vi "GxSingleCam.vi"() -> ()   [LabVIEW 2013]
uses:
  GxLVLib/GxLVlib.lvlib
  F:/GxILibrary/Labview/trunk/private/dev/src/C#/x86/GxLVLib/dll/GxIAPINET.dll
  private/dev/src/C#/x86/GxLVLib/dll/GxIAPINET.dll
  <vilib>/vision/Image Controls.llb/IMAQ Image.ctl
panel:
  out "Image":T1(plugin-control)
  out "是否退出":bool
  in  "图片存储路径":path
  in  "保存图片":bool
  in  "Image Src":T1
  out "采集回调":refnum<k27>
  out "是否支持白平衡":bool
  out "采集状态":bool
  out "设备状态":bool
  in  "IGxFactory":refnum<k24>
  in  "安全退出":bool
  in  "IGxStream":refnum<k24>
  in  "IGxDevice":refnum<k24>
  out "error out":errorcluster
  in  "发送软触发":bool
  in  "自动白平衡":string(combo)
  in  "增益":dbl format="%#_6f"
  in  "曝光时间":dbl
  in  "触发源":string(combo)
  in  "触发模式":string(combo)
  in  "停止采集":bool
  in  "开始采集":bool
  in  "关闭设备":bool
  in  "打开设备":bool
  # "触发模式"
  # "触发源"
  # "软触发"
  # "曝光时间(us)"
  # "增益(dB)"
  # "自动白平衡"
  # "保存图片"
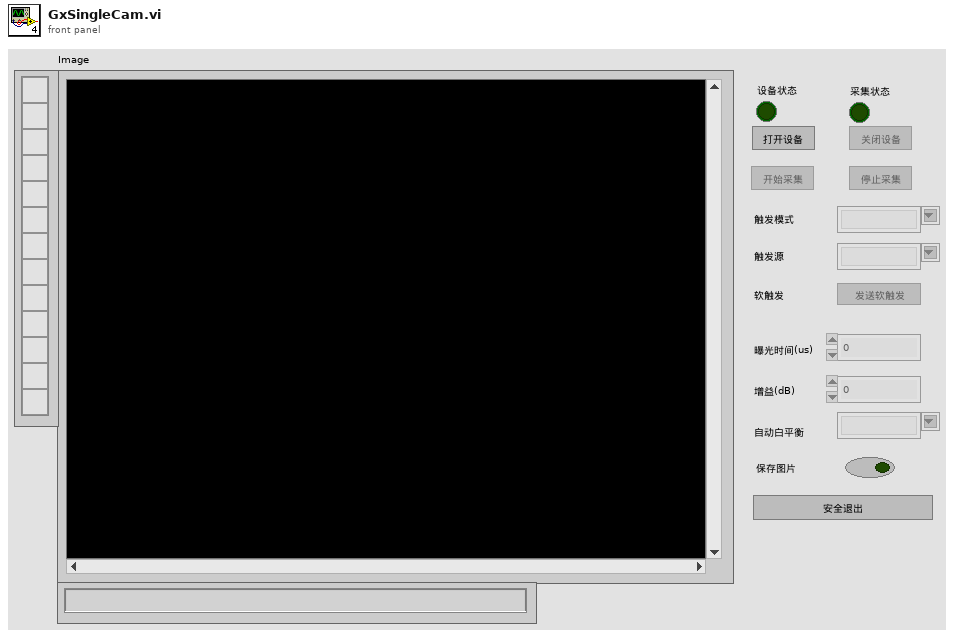
[diagram p1: front panel]
types:
  T1 = typedef "IMAQ Image.ctl" = refnum<image>
  T2 = typedef "Semaphore RefNum" = refnum<k1>
  T3 = enum8{"Enabled", "Disabled", "Disabled and Grayed Out"}
  T4 = typedef "Image Type" = u32
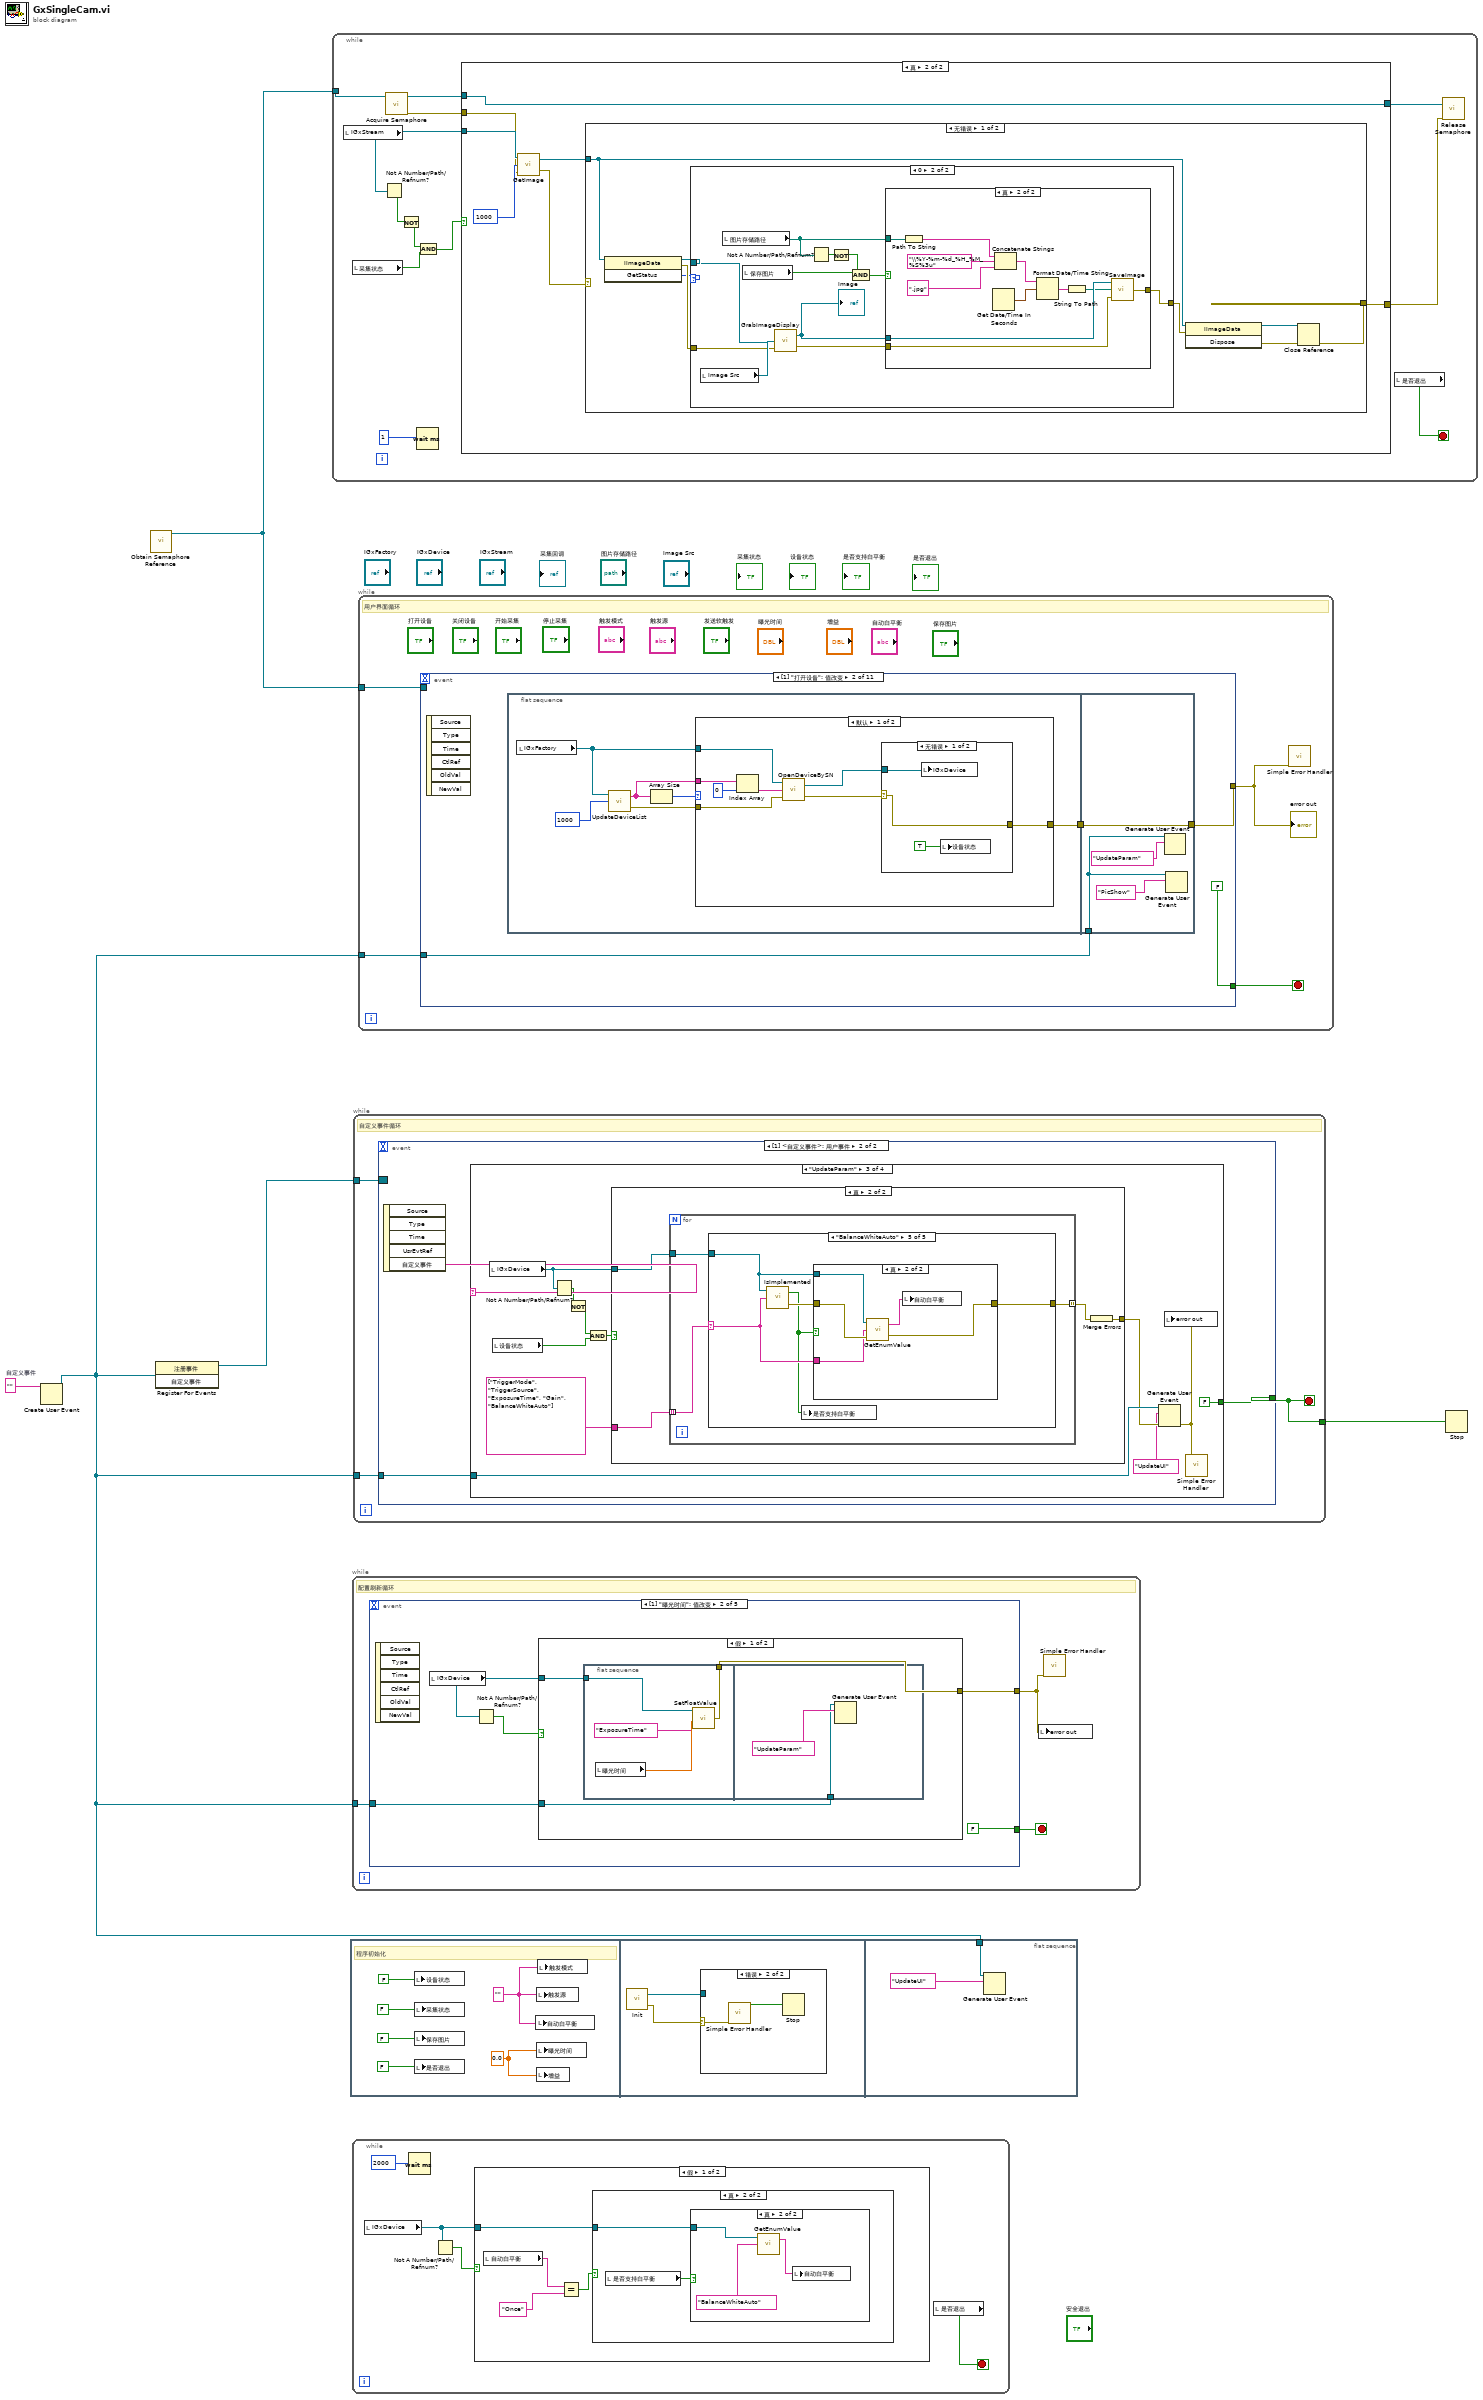
[diagram p0: block diagram]
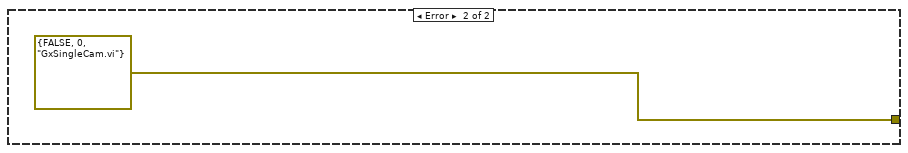
[diagram p5: hidden frame]
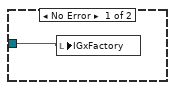
[diagram p9: hidden frame]
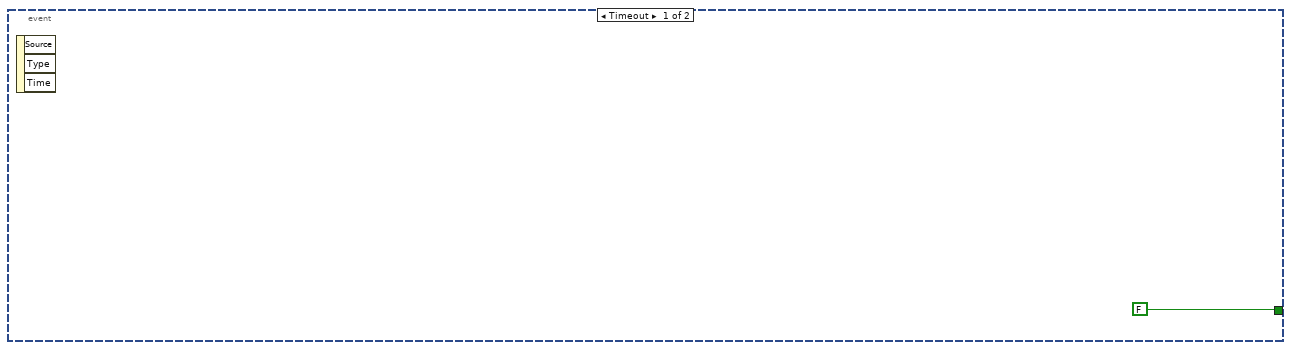
[diagram p10: hidden frame]
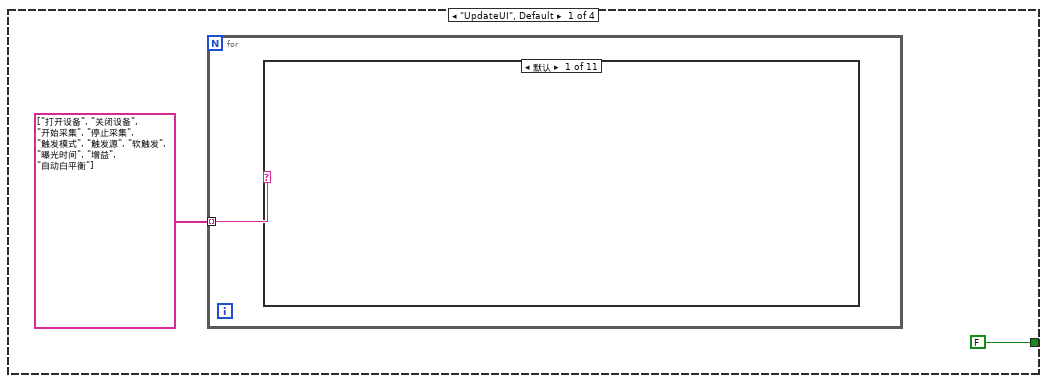
[diagram p11: hidden frame]
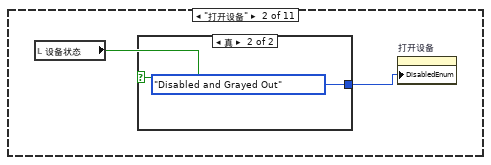
[diagram p12: hidden frame]
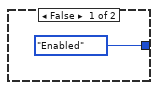
[diagram p13: hidden frame]
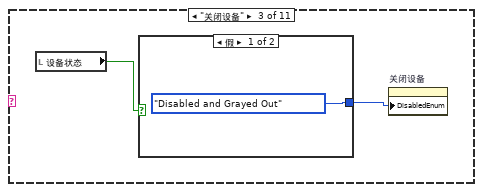
[diagram p14: hidden frame]
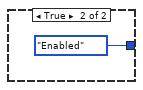
[diagram p15: hidden frame]
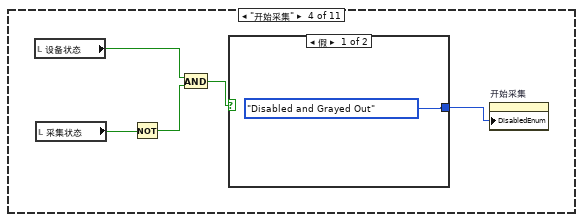
[diagram p16: hidden frame]
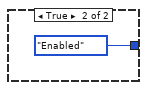
[diagram p17: hidden frame]
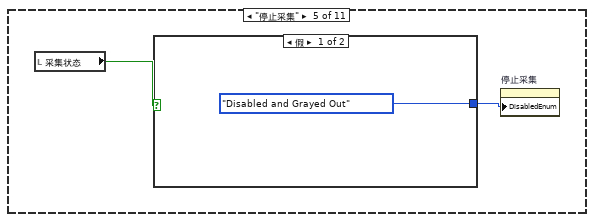
[diagram p18: hidden frame]
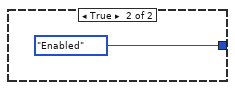
[diagram p19: hidden frame]
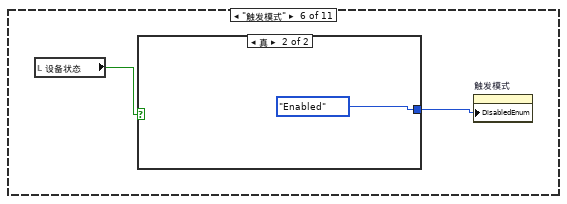
[diagram p20: hidden frame]
diagram:
  w5 = ""  # 自定义事件
  n1 = Create User Event(user event datatype=w5) -> (user event=w2:refnum<user-event>)  [unwired: 1 in, 1 out]
  n2 = call <vilib>:"Obtain Semaphore Reference.vi"() -> ("semaphore"=w1:T2)  [unwired: 5 in, 2 out]
  n3 = register-events(w2) -> (reference out=w4:refnum<event-registration>)  [unwired: 2 in, 1 out]
  n4 = while {
    tunnel: w1 -> [w10]
    stop <- w17 stop-if-true
    n5 = local read "IGxStream"() -> (w16:refnum<k24>)
    n6 = local read "采集状态"() -> (w13:bool)
    n7 = Not A Number/Path/Refnum?(number/path/refnum=w16) -> (NaN/Path/Refnum?=w15:bool)
    n8 = call <vilib>:"Acquire Semaphore.vi"("semaphore"=w10) -> ("error out"=w7:errorcluster, "semaphore out"=w9:T2)  [unwired: 4 in, 1 out]
    n9 = Not(x=w15) -> (.not. x?=w14:bool)
    n10 = Wait (ms)(milliseconds to wait=1) -> ()  [unwired: 1 out]
    n11 = And(x=w14, y=w13) -> (x .and. y?=w12:bool)
    n12 = case shown="真" w12 {
      tunnel: w16 -> [_ w26]
      tunnel: [w18 w24] -> w8
      tunnel: w9 -> [w18 w24]
      tunnel: w7 -> [w19 w23]
      tunnel: [w19 w20] -> w6
      frame False {
      }
      frame True {
        n13 = call "GetImage.vi"("error in (no error)"=w23, "Time out"=1000, "IGxStream"=w26) -> ("error out"=w22:errorcluster, "IImageData"=w21:refnum<k24>)
        n14 = case shown="无错误" w22 {
          tunnel: w21 -> [w30 _]
          tunnel: [w28 errorcluster {FALSE, 0, "GxSingleCam.vi"}] -> w20
          frame No Error {
            n15 = invoke class="IImageData" method="GetStatus"(reference=w30) -> (reference out=w33:refnum<k24>, error out=w34:errorcluster, "GetStatus"=w32:i32)  [unwired: 2 in]
            n16 = case shown="0" w32 {
              tunnel: [w35 w40] -> w31
              tunnel: w33 -> [_ w37]
              tunnel: w34 -> [w35 w38]
              frame Default {
              }
              frame 0 {
                n17 = local read "Image Src"() -> (w41:T1)
                n18 = local read "图片存储路径"() -> (w39:path)
                n19 = local read "保存图片"() -> (w44:bool)
                n20 = call "GrabImageDisplay.vi"("error in (no error)"=w38, "Image Src"=w41, "IBaseData"=w37) -> ("error out"=w46:errorcluster, "Image out"=w36:T1)
                "Image" <- w36
                n21 = Not A Number/Path/Refnum?(number/path/refnum=w39) -> (NaN/Path/Refnum?=w42:bool)
                n22 = Not(x=w42) -> (.not. x?=w43:bool)
                n23 = And(x=w44, y=w43) -> (x .and. y?=w45:bool)
                n24 = case shown="真" w45 {
                  tunnel: w39 -> [_ w54]
                  tunnel: w36 -> [_ w53]
                  tunnel: w46 -> [w47 w51]
                  tunnel: [w47 w50] -> w40
                  frame False {
                  }
                  frame True {
                    n25 = Path To String(path=w54) -> (string=w55:string)
                    n26 = Get Date/Time In Seconds() -> (seconds since 1Jan1904=w57:timestamp)
                    n27 = Concatenate Strings(w55, "\\%Y-%m-%d_%H_%M_%S%3u", ".jpg") -> (w56:string)
                    n28 = Format Date/Time String(time format string (%c)=w56, seconds (now)=w57) -> (date/time string=w58:string)  [unwired: 1 in]
                    n29 = String To Path(string=w58) -> (path=w52:path)
                    n30 = call "SaveImage.vi"("error in (no error)"=w51, "Path"=w52, "Image Src"=w53) -> ("error out"=w50:errorcluster)
                  }
                }
              }
            }
            n31 = invoke class="IImageData" method="Dispose"(reference=w30, error in=w31) -> (reference out=w27:refnum<k24>, error out=w29:errorcluster)  [unwired: 1 in, 1 out]
            n32 = Close Reference(reference=w27, error in (no error)=w29) -> (error out=w28:errorcluster)
          }
          frame Error {
          }
        }
      }
    }
    n33 = local read "是否退出"() -> (w17:bool)
    n34 = call <vilib>:"Release Semaphore.vi"("error in (no error)"=w6, "semaphore"=w8) -> ()  [unwired: 4 in, 2 out]
  }
  n35 = flat-sequence {
    tunnel: w2 -> [w71]
    frame #0 {
      w62 = 0.0
      w63 = ""
      # "程序初始化"
      n36 = local write "设备状态"(FALSE) -> ()
      n37 = local write "采集状态"(FALSE) -> ()
      n38 = local write "保存图片"(FALSE) -> ()
      n39 = local write "是否退出"(FALSE) -> ()
      n40 = local write "自动白平衡"(w63) -> ()
      n41 = local write "触发源"(w63) -> ()
      n42 = local write "曝光时间"(w62) -> ()
      n43 = local write "增益"(w62) -> ()
      n44 = local write "触发模式"(w63) -> ()
    }
    frame #1 {
      n45 = call "Init.vi"() -> ("IGxFactory"=w67:refnum<k24>, "error out"=w66:errorcluster)  [unwired: 1 in]
      n46 = case shown="错误" w66 {
        selector: w66 -> [_ w69]
        tunnel: w67 -> [w68 _]
        frame No Error {
          n47 = local write "IGxFactory"(w68) -> ()
        }
        frame Error {
          n48 = call <vilib>:"Simple Error Handler.vi"("error in (no error)"=w69) -> ("error?"=w70:bool)  [unwired: 4 in, 4 out]
          n49 = Stop(stop? (T)=w70) -> ()
        }
      }
    }
    frame #2 {
      n50 = Generate User Event(user event=w71, event data cluster="UpdateUI") -> ()  [unwired: 2 in, 2 out]
    }
  }
  n51 = while {
    tunnel: w2 -> [w73]
    stop <- w75 stop-if-true
    # "配置刷新循环"
    n52 = event shown="[1] \"曝光时间\": 值改变" {
      selector: _ -> [_ _ _ _ _]
      dyn-events: _ -> [_ _ _ _ _]
      timeout: _ -> [_ _ _ _ _]
      tunnel: [errorcluster {FALSE, 0, ""} w80 w95 w110 errorcluster {"status"=FALSE, "code"=0, "source"=""} ("错误常量")] -> w74
      tunnel: [FALSE FALSE FALSE FALSE TRUE] -> w75
      tunnel: w73 -> [_ w78 w93 w108 _]
      event Timeout {
        n53 = event-data() -> ()  [unwired: 1 in, 3 out]
      }
      event "曝光时间": Value Change {
        n54 = event-data() -> ()  [unwired: 1 in, 6 out]
        n55 = local read "IGxDevice"() -> (w81:refnum<k24>)
        n56 = Not A Number/Path/Refnum?(number/path/refnum=w81) -> (NaN/Path/Refnum?=w82:bool)
        n57 = case shown="假" w82 {
          tunnel: w81 -> [w85 _]
          tunnel: [w84 errorcluster {TRUE, 5000, "GxSingleCam.vi"}] -> w80
          tunnel: w78 -> [w83 _]
          frame False {
            n58 = flat-sequence {
              tunnel: w85 -> [w87]
              tunnel: [w86] -> w84
              tunnel: w83 -> [w90]
              frame #0 {
                n59 = local read "曝光时间"() -> (w89:dbl)
                n60 = call "SetFloatValue.vi"("Float Value"=w89, "Feature Name"="ExposureTime", "IGxDevice"=w87) -> ("error out"=w86:errorcluster)  [unwired: 1 in]
              }
              frame #1 {
                n61 = Generate User Event(user event=w90, event data cluster="UpdateParam") -> ()  [unwired: 2 in, 2 out]
              }
            }
          }
          frame True {
          }
        }
      }
      event "增益": Value Change {
        n62 = event-data() -> ()  [unwired: 1 in, 6 out]
        n63 = local read "IGxDevice"() -> (w97:refnum<k24>)
        n64 = Not A Number/Path/Refnum?(number/path/refnum=w97) -> (NaN/Path/Refnum?=w96:bool)
        n65 = case shown="真" w96 {
          tunnel: w97 -> [w100 _]
          tunnel: [w99 errorcluster {TRUE, 0, "设备句柄无效"}] -> w95
          tunnel: w93 -> [w98 _]
          frame False {
            n66 = flat-sequence {
              tunnel: w100 -> [w102]
              tunnel: [w101] -> w99
              tunnel: w98 -> [w106]
              frame #0 {
                n67 = local read "增益"() -> (w104:dbl)
                n68 = call "SetFloatValue.vi"("Float Value"=w104, "Feature Name"="Gain", "IGxDevice"=w102) -> ("error out"=w101:errorcluster)  [unwired: 1 in]
              }
              frame #1 {
                n69 = Generate User Event(user event=w106, event data cluster="UpdateParam") -> ()  [unwired: 2 in, 2 out]
              }
            }
          }
          frame True {
          }
        }
      }
      event "自动白平衡": Value Change {
        n70 = event-data() -> ()  [unwired: 1 in, 6 out]
        n71 = local read "IGxDevice"() -> (w111:refnum<k24>)
        n72 = Not A Number/Path/Refnum?(number/path/refnum=w111) -> (NaN/Path/Refnum?=w112:bool)
        n73 = case shown="假" w112 {
          tunnel: w111 -> [w115 _]
          tunnel: [w114 errorcluster {TRUE, 0, "设备句柄无效"}] -> w110
          tunnel: w108 -> [w113 _]
          frame False {
            n74 = flat-sequence {
              tunnel: w115 -> [w117]
              tunnel: [w116] -> w114
              tunnel: w113 -> [w120]
              frame #0 {
                n75 = local read "自动白平衡"() -> (w119:string)
                n76 = call "SetEnumValue.vi"("Enum Value"=w119, "Feature Name"="BalanceWhiteAuto", "IGxDevice"=w117) -> ("error out"=w116:errorcluster)  [unwired: 1 in]
              }
              frame #1 {
                n77 = Generate User Event(user event=w120, event data cluster="UpdateParam") -> ()  [unwired: 2 in, 2 out]
              }
            }
          }
          frame True {
          }
        }
      }
      event "安全退出": Value Change {
        n78 = event-data() -> ()  [unwired: 1 in, 6 out]
      }
    }
    n79 = local write "error out"(w74) -> ()
    n80 = call <vilib>:"Simple Error Handler.vi"("error in (no error)"=w74) -> ()  [unwired: 4 in, 5 out]
  }
  n81 = while {
    stop <- w125 stop-if-true
    n82 = local read "IGxDevice"() -> (w127:refnum<k24>)
    n83 = Wait (ms)(milliseconds to wait=2000) -> ()  [unwired: 1 out]
    n84 = Not A Number/Path/Refnum?(number/path/refnum=w127) -> (NaN/Path/Refnum?=w126:bool)
    n85 = case shown="假" w126 {
      tunnel: w127 -> [w132 _]
      frame False {
        n86 = local read "自动白平衡"() -> (w130:string)
        n87 = Equal?(x=w130, y="Once") -> (x = y?=w129:bool)
        n88 = case shown="真" w129 {
          tunnel: w132 -> [_ w133]
          frame False {
          }
          frame True {
            n89 = local read "是否支持白平衡"() -> (w134:bool)
            n90 = case shown="真" w134 {
              tunnel: w133 -> [_ w137]
              frame False {
              }
              frame True {
                n91 = call "GetEnumValue.vi"("Feature Name"="BalanceWhiteAuto", "IGxDevice"=w137) -> ("Enum Value"=w135:string)  [unwired: 1 in, 1 out]
                n92 = local write "自动白平衡"(w135) -> ()
              }
            }
          }
        }
      }
      frame True {
      }
    }
    n93 = local read "是否退出"() -> (w125:bool)
  }
  n94 = while {
    tunnel: w4 -> [w140]
    tunnel: w2 -> [w139]
    tunnel: [w138] -> w3
    stop <- w138 stop-if-true
    # "自定义事件循环"
    n95 = event shown="[1] <自定义事件>: 用户事件" {
      selector: w140 -> [_ _]
      dyn-events: _ -> [_ _]
      timeout: _ -> [_ _]
      tunnel: [FALSE w142] -> w138
      tunnel: w139 -> [_ w143]
      event Timeout {
        n96 = event-data() -> ()  [unwired: 1 in, 3 out]
      }
      event User Event {
        n97 = event-data() -> ("自定义事件"=w144:string)  [unwired: 1 in, 4 out]
        n98 = case shown="\"UpdateParam\"" w144 {
          tunnel: w143 -> [_ _ w275 _]
          tunnel: [FALSE TRUE FALSE FALSE] -> w142
          frame "UpdateUI", Default {
            n99 = for {
              tunnel: string[] ["打开设备", "关闭设备", "开始采集", "停止采集", "触发模式", "触发源", "软触发", "曝光时间", "增益", "自动白平衡"] -> [w147] mode=indexing
              n100 = case shown="默认" w147 {
                frame Default {
                }
                frame "打开设备" {
                  n101 = local read "设备状态"() -> (w149:bool)
                  n102 = case shown="真" w149 {
                    tunnel: [T3."Enabled" ("禁用") T3."Disabled and Grayed Out" ("禁用")] -> w148
                    frame False {
                    }
                    frame True {
                    }
                  }
                  n103 = property on="打开设备" class="Bool"("DisabledEnum"=w148) -> ()  [unwired: 2 in, 2 out]
                }
                frame "关闭设备" {
                  n104 = local read "设备状态"() -> (w153:bool)
                  n105 = case shown="假" w153 {
                    tunnel: [T3."Disabled and Grayed Out" ("禁用") T3."Enabled" ("禁用")] -> w152
                    frame False {
                    }
                    frame True {
                    }
                  }
                  n106 = property on="关闭设备" class="Bool"("DisabledEnum"=w152) -> ()  [unwired: 2 in, 2 out]
                }
                frame "开始采集" {
                  n107 = local read "设备状态"() -> (w159:bool)
                  n108 = local read "采集状态"() -> (w160:bool)
                  n109 = Not(x=w160) -> (.not. x?=w158:bool)
                  n110 = And(x=w159, y=w158) -> (x .and. y?=w157:bool)
                  n111 = case shown="假" w157 {
                    tunnel: [T3."Disabled and Grayed Out" ("禁用") T3."Enabled" ("禁用")] -> w156
                    frame False {
                    }
                    frame True {
                    }
                  }
                  n112 = property on="开始采集" class="Bool"("DisabledEnum"=w156) -> ()  [unwired: 2 in, 2 out]
                }
                frame "停止采集" {
                  n113 = local read "采集状态"() -> (w164:bool)
                  n114 = case shown="假" w164 {
                    tunnel: [T3."Disabled and Grayed Out" ("禁用") T3."Enabled" ("禁用")] -> w163
                    frame False {
                    }
                    frame True {
                    }
                  }
                  n115 = property on="停止采集" class="Bool"("DisabledEnum"=w163) -> ()  [unwired: 2 in, 2 out]
                }
                frame "触发模式" {
                  n116 = local read "设备状态"() -> (w168:bool)
                  n117 = case shown="真" w168 {
                    tunnel: [T3."Disabled and Grayed Out" ("禁用") T3."Enabled" ("禁用")] -> w167
                    frame False {
                    }
                    frame True {
                    }
                  }
                  n118 = property on="触发模式" class="CmbBox"("DisabledEnum"=w167) -> ()  [unwired: 2 in, 2 out]
                }
                frame "触发源" {
                  n119 = local read "设备状态"() -> (w174:bool)
                  n120 = local read "触发模式"() -> (w176:string)
                  n121 = Equal?(x=w176, y="On") -> (x = y?=w173:bool)
                  n122 = And(x=w174, y=w173) -> (x .and. y?=w172:bool)
                  n123 = case shown="假" w172 {
                    tunnel: [T3."Disabled and Grayed Out" ("禁用") T3."Enabled" ("禁用")] -> w171
                    frame False {
                    }
                    frame True {
                    }
                  }
                  n124 = property on="触发源" class="CmbBox"("DisabledEnum"=w171) -> ()  [unwired: 2 in, 2 out]
                }
                frame "软触发" {
                  n125 = local read "设备状态"() -> (w181:bool)
                  n126 = local read "采集状态"() -> (w180:bool)
                  n127 = local read "触发模式"() -> (w190:string)
                  n128 = local read "触发源"() -> (w188:string)
                  n129 = Equal?(x=w190, y="On") -> (x = y?=w186:bool)
                  n130 = Equal?(x=w188, y="Software") -> (x = y?=w185:bool)
                  n131 = And(x=w181, y=w180) -> (x .and. y?=w179:bool)
                  n132 = And(x=w186, y=w185) -> (x .and. y?=w184:bool)
                  n133 = And(x=w179, y=w184) -> (x .and. y?=w183:bool)
                  n134 = case shown="真" w183 {
                    tunnel: [T3."Disabled and Grayed Out" ("禁用") T3."Enabled" ("禁用")] -> w182
                    frame False {
                    }
                    frame True {
                    }
                  }
                  n135 = property on="发送软触发" class="Bool"("DisabledEnum"=w182) -> ()  [unwired: 2 in, 2 out]
                }
                frame "曝光时间" {
                  n136 = local read "设备状态"() -> (w194:bool)
                  n137 = case shown="假" w194 {
                    tunnel: [T3."Disabled and Grayed Out" ("禁用") T3."Enabled" ("禁用")] -> w193
                    frame False {
                    }
                    frame True {
                    }
                  }
                  n138 = property on="曝光时间" class="DigNum (严格)"("DisabledEnum"=w193) -> ()  [unwired: 2 in, 2 out]
                }
                frame "增益" {
                  n139 = local read "设备状态"() -> (w198:bool)
                  n140 = case shown="真" w198 {
                    tunnel: [T3."Disabled and Grayed Out" ("禁用") T3."Enabled" ("禁用")] -> w197
                    frame False {
                    }
                    frame True {
                    }
                  }
                  n141 = property on="增益" class="DigNum (严格)"("DisabledEnum"=w197) -> ()  [unwired: 2 in, 2 out]
                }
                frame "自动白平衡" {
                  n142 = local read "是否支持白平衡"() -> (w204:bool)
                  n143 = local read "设备状态"() -> (w203:bool)
                  n144 = And(x=w203, y=w204) -> (x .and. y?=w202:bool)
                  n145 = case shown="真" w202 {
                    tunnel: [T3."Disabled and Grayed Out" ("禁用") T3."Enabled" ("禁用")] -> w201
                    frame False {
                    }
                    frame True {
                    }
                  }
                  n146 = property on="自动白平衡" class="CmbBox"("DisabledEnum"=w201) -> ()  [unwired: 2 in, 2 out]
                }
              }
            }
          }
          frame "Quit" {
            n147 = for {
              tunnel: string[] ["打开设备", "关闭设备", "开始采集", "停止采集", "触发模式", "触发源", "软触发", "曝光时间", "增益", "自动白平衡"] -> [w211] mode=indexing
              n148 = case shown="\"停止采集\"" w211 {
                frame Default {
                }
                frame "打开设备" {
                  n149 = local read "设备状态"() -> (w213:bool)
                  n150 = case shown="真" w213 {
                    tunnel: [T3."Enabled" ("禁用") T3."Disabled and Grayed Out" ("禁用")] -> w212
                    frame False {
                    }
                    frame True {
                    }
                  }
                  n151 = property on="打开设备" class="Bool"("DisabledEnum"=w212) -> ()  [unwired: 2 in, 2 out]
                }
                frame "关闭设备" {
                  n152 = local read "设备状态"() -> (w217:bool)
                  n153 = case shown="假" w217 {
                    tunnel: [T3."Disabled and Grayed Out" ("禁用") T3."Enabled" ("禁用")] -> w216
                    frame False {
                    }
                    frame True {
                    }
                  }
                  n154 = property on="关闭设备" class="Bool"("DisabledEnum"=w216) -> ()  [unwired: 2 in, 2 out]
                }
                frame "开始采集" {
                  n155 = local read "设备状态"() -> (w223:bool)
                  n156 = local read "采集状态"() -> (w224:bool)
                  n157 = Not(x=w224) -> (.not. x?=w222:bool)
                  n158 = And(x=w223, y=w222) -> (x .and. y?=w221:bool)
                  n159 = case shown="假" w221 {
                    tunnel: [T3."Disabled and Grayed Out" ("禁用") T3."Enabled" ("禁用")] -> w220
                    frame False {
                    }
                    frame True {
                    }
                  }
                  n160 = property on="开始采集" class="Bool"("DisabledEnum"=w220) -> ()  [unwired: 2 in, 2 out]
                }
                frame "停止采集" {
                  n161 = local read "采集状态"() -> (w228:bool)
                  n162 = case shown="假" w228 {
                    tunnel: [T3."Disabled and Grayed Out" ("禁用") T3."Enabled" ("禁用")] -> w227
                    frame False {
                    }
                    frame True {
                    }
                  }
                  n163 = property on="停止采集" class="Bool"("DisabledEnum"=w227) -> ()  [unwired: 2 in, 2 out]
                }
                frame "触发模式" {
                  n164 = local read "设备状态"() -> (w232:bool)
                  n165 = case shown="真" w232 {
                    tunnel: [T3."Disabled and Grayed Out" ("禁用") T3."Enabled" ("禁用")] -> w231
                    frame False {
                    }
                    frame True {
                    }
                  }
                  n166 = property on="触发模式" class="CmbBox"("DisabledEnum"=w231) -> ()  [unwired: 2 in, 2 out]
                }
                frame "触发源" {
                  n167 = local read "设备状态"() -> (w238:bool)
                  n168 = local read "触发模式"() -> (w240:string)
                  n169 = Equal?(x=w240, y="On") -> (x = y?=w237:bool)
                  n170 = And(x=w238, y=w237) -> (x .and. y?=w236:bool)
                  n171 = case shown="假" w236 {
                    tunnel: [T3."Disabled and Grayed Out" ("禁用") T3."Enabled" ("禁用")] -> w235
                    frame False {
                    }
                    frame True {
                    }
                  }
                  n172 = property on="触发源" class="CmbBox"("DisabledEnum"=w235) -> ()  [unwired: 2 in, 2 out]
                }
                frame "软触发" {
                  n173 = local read "设备状态"() -> (w245:bool)
                  n174 = local read "采集状态"() -> (w244:bool)
                  n175 = local read "触发模式"() -> (w254:string)
                  n176 = local read "触发源"() -> (w252:string)
                  n177 = Equal?(x=w254, y="On") -> (x = y?=w250:bool)
                  n178 = Equal?(x=w252, y="Software") -> (x = y?=w249:bool)
                  n179 = And(x=w245, y=w244) -> (x .and. y?=w243:bool)
                  n180 = And(x=w250, y=w249) -> (x .and. y?=w248:bool)
                  n181 = And(x=w243, y=w248) -> (x .and. y?=w247:bool)
                  n182 = case shown="真" w247 {
                    tunnel: [T3."Disabled and Grayed Out" ("禁用") T3."Enabled" ("禁用")] -> w246
                    frame False {
                    }
                    frame True {
                    }
                  }
                  n183 = property on="发送软触发" class="Bool"("DisabledEnum"=w246) -> ()  [unwired: 2 in, 2 out]
                }
                frame "曝光时间" {
                  n184 = local read "设备状态"() -> (w258:bool)
                  n185 = case shown="假" w258 {
                    tunnel: [T3."Disabled and Grayed Out" ("禁用") T3."Enabled" ("禁用")] -> w257
                    frame False {
                    }
                    frame True {
                    }
                  }
                  n186 = property on="曝光时间" class="DigNum (严格)"("DisabledEnum"=w257) -> ()  [unwired: 2 in, 2 out]
                }
                frame "增益" {
                  n187 = local read "设备状态"() -> (w262:bool)
                  n188 = case shown="真" w262 {
                    tunnel: [T3."Disabled and Grayed Out" ("禁用") T3."Enabled" ("禁用")] -> w261
                    frame False {
                    }
                    frame True {
                    }
                  }
                  n189 = property on="增益" class="DigNum (严格)"("DisabledEnum"=w261) -> ()  [unwired: 2 in, 2 out]
                }
                frame "自动白平衡" {
                  n190 = local read "是否支持白平衡"() -> (w268:bool)
                  n191 = local read "设备状态"() -> (w267:bool)
                  n192 = And(x=w267, y=w268) -> (x .and. y?=w266:bool)
                  n193 = case shown="真" w266 {
                    tunnel: [T3."Disabled and Grayed Out" ("禁用") T3."Enabled" ("禁用")] -> w265
                    frame False {
                    }
                    frame True {
                    }
                  }
                  n194 = property on="自动白平衡" class="CmbBox"("DisabledEnum"=w265) -> ()  [unwired: 2 in, 2 out]
                }
              }
            }
            n195 = local read "IGxFactory"() -> (w207:refnum<k24>)
            n196 = call "UnInit.vi"("IGxFactory"=w207) -> ("error out"=w208:errorcluster)  [unwired: 1 in]
            n197 = Close Reference(reference=w207, error in (no error)=w208) -> ()  [unwired: 1 out]
          }
          frame "UpdateParam" {
            n198 = local read "IGxDevice"() -> (w277:refnum<k24>)
            n199 = local read "设备状态"() -> (w281:bool)
            n200 = Not A Number/Path/Refnum?(number/path/refnum=w277) -> (NaN/Path/Refnum?=w278:bool)
            n201 = Not(x=w278) -> (.not. x?=w280:bool)
            n202 = And(x=w280, y=w281) -> (x .and. y?=w279:bool)
            n203 = case shown="真" w279 {
              tunnel: [errorcluster {FALSE, 0, ""} w283] -> w274
              tunnel: string[] ["TriggerMode", "TriggerSource", "ExposureTime", "Gain", "BalanceWhiteAuto"] -> [_ w286]
              tunnel: w277 -> [_ w285]
              frame False {
              }
              frame True {
                n204 = for {
                  tunnel: w286 -> [w289] mode=indexing
                  tunnel: w285 -> [w288]
                  tunnel: [w287] -> w284 mode=indexing
                  n205 = case shown="\"BalanceWhiteAuto\"" w289 {
                    selector: w289 -> [w292 w296 w300 w304 w307]
                    tunnel: w288 -> [w293 w297 w301 w305 w308]
                    tunnel: [w290 w294 w298 w302 w310] -> w287
                    frame "TriggerMode", Default {
                      n206 = call "GetEnumValue.vi"("Feature Name"=w292, "IGxDevice"=w293) -> ("error out"=w290:errorcluster, "Enum Value"=w291:string)  [unwired: 1 in]
                      n207 = local write "触发模式"(w291) -> ()
                    }
                    frame "TriggerSource" {
                      n208 = call "GetEnumValue.vi"("Feature Name"=w296, "IGxDevice"=w297) -> ("error out"=w294:errorcluster, "Enum Value"=w295:string)  [unwired: 1 in]
                      n209 = local write "触发源"(w295) -> ()
                    }
                    frame "ExposureTime" {
                      n210 = call "GetFloatValue.vi"("Feature Name"=w300, "IGxDevice"=w301) -> ("error out"=w298:errorcluster, "Float Value"=w299:dbl)  [unwired: 1 in]
                      n211 = local write "曝光时间"(w299) -> ()
                    }
                    frame "Gain" {
                      n212 = call "GetFloatValue.vi"("Feature Name"=w304, "IGxDevice"=w305) -> ("error out"=w302:errorcluster, "Float Value"=w303:dbl)  [unwired: 1 in]
                      n213 = local write "增益"(w303) -> ()
                    }
                    frame "BalanceWhiteAuto" {
                      n214 = call "IsImplemented.vi"("Feature Name"=w307, "IGxDevice"=w308) -> ("error out"=w309:errorcluster, "IsImplement"=w306:bool)  [unwired: 1 in]
                      n215 = local write "是否支持白平衡"(w306) -> ()
                      n216 = case shown="真" w306 {
                        tunnel: [w311 w315] -> w310
                        tunnel: w309 -> [w311 w316]
                        tunnel: w308 -> [_ w313]
                        tunnel: w307 -> [_ w312]
                        frame False {
                        }
                        frame True {
                          n217 = call "GetEnumValue.vi"("error in (no error)"=w316, "Feature Name"=w312, "IGxDevice"=w313) -> ("error out"=w315:errorcluster, "Enum Value"=w314:string)
                          n218 = local write "自动白平衡"(w314) -> ()
                        }
                      }
                    }
                  }
                }
                n219 = Merge Errors(w284) -> (w283:errorcluster)
              }
            }
            n220 = Generate User Event(user event=w275, event data cluster="UpdateUI", error in=w274) -> (error out=w273:errorcluster)  [unwired: 1 in, 1 out]
            n221 = local write "error out"(w273) -> ()
            n222 = call <vilib>:"Simple Error Handler.vi"("error in (no error)"=w273) -> ()  [unwired: 4 in, 5 out]
          }
          frame "PicShow" {
            n223 = local read "IGxDevice"() -> (w319:refnum<k24>)
            n224 = local read "设备状态"() -> (w323:bool)
            n225 = Not A Number/Path/Refnum?(number/path/refnum=w319) -> (NaN/Path/Refnum?=w320:bool)
            n226 = Not(x=w320) -> (.not. x?=w322:bool)
            n227 = And(x=w322, y=w323) -> (x .and. y?=w321:bool)
            n228 = case shown="真" w321 {
              tunnel: [errorcluster {FALSE, 0, ""} errorcluster {FALSE, 0, ""}] -> w317
              tunnel: w319 -> [_ w329]
              frame False {
              }
              frame True {
                n229 = call "IsImplemented.vi"("Feature Name"="PixelColorFilter", "IGxDevice"=w329) -> ("IsImplement"=w331:bool)  [unwired: 1 in, 1 out]
                n230 = case shown="真" w331 {
                  tunnel: w329 -> [_ w338]
                  tunnel: [w332 w333] -> w326
                  frame False {
                    w332 = T4 0 items=["Grayscale (U8)", "Grayscale (I16)", "Grayscale (SGL)", "Complex (CSG)", "RGB (U32)", "HSL (U32)", "RGB (U64)", "Grayscale (U16)"] ("Image Type")
                  }
                  frame True {
                    n231 = call "GetEnumValue.vi"("Feature Name"="PixelColorFilter", "IGxDevice"=w338) -> ("Enum Value"=w336:string)  [unwired: 1 in, 1 out]
                    n232 = Equal?(x=w336, y="None") -> (x = y?=w334:bool)
                    n233 = case shown="假" w334 {
                      tunnel: [w339 w340] -> w333
                      frame False {
                        w339 = T4 4 items=["Grayscale (U8)", "Grayscale (I16)", "Grayscale (SGL)", "Complex (CSG)", "RGB (U32)", "HSL (U32)", "RGB (U64)", "Grayscale (U16)"] ("Image Type")
                      }
                      frame True {
                        w340 = T4 0 items=["Grayscale (U8)", "Grayscale (I16)", "Grayscale (SGL)", "Complex (CSG)", "RGB (U32)", "HSL (U32)", "RGB (U64)", "Grayscale (U16)"] ("Image Type")
                      }
                    }
                  }
                }
                n234 = call "IMAQ Create"("Image Name"="", "Image Type"=w326) -> ("New Image"=w327:T1)  [unwired: 3 in, 1 out]
                n235 = local write "Image Src"(w327) -> ()
              }
            }
            n236 = local write "error out"(w317) -> ()
            n237 = call <vilib>:"Simple Error Handler.vi"("error in (no error)"=w317) -> ()  [unwired: 4 in, 5 out]
          }
        }
      }
    }
  }
  n238 = while {
    tunnel: w2 -> [w344]
    tunnel: w1 -> [w341]
    stop <- w342 stop-if-true
    # "用户界面循环"
    n239 = event shown="[1] \"打开设备\": 值改变" {
      selector: _ -> [_ _ _ _ _ _ _ _ _ _ _]
      dyn-events: _ -> [_ _ _ _ _ _ _ _ _ _ _]
      timeout: _ -> [_ _ _ _ _ _ _ _ _ _ _]
      tunnel: [errorcluster {FALSE, 0, ""} w349 _ w410 w429 w452 w460 w467 _ _ _] -> w343
      tunnel: [FALSE FALSE FALSE FALSE FALSE FALSE FALSE FALSE FALSE TRUE TRUE] -> w342
      tunnel: w344 -> [_ w347 w377 w408 w430 w454 w461 w469 _ w487 w520]
      tunnel: w341 -> [_ _ w376 _ w436 _ _ _ _ w486 w519]
      event Timeout {
        n240 = event-data() -> ()  [unwired: 1 in, 3 out]
      }
      event "打开设备": Value Change {
        n241 = event-data() -> ()  [unwired: 1 in, 6 out]
        n242 = flat-sequence {
          tunnel: [w353] -> w348
          tunnel: [w375] -> w349
          tunnel: w348 -> [w375]
          tunnel: w347 -> [w372]
          frame #0 {
            n243 = local read "IGxFactory"() -> (w354:refnum<k24>)
            n244 = call "UpdateDeviceList.vi"("time out"=1000, "IGxFactory"=w354) -> ("error out"=w351:errorcluster, "DeviceSNList"=w352:string[])  [unwired: 1 in]
            n245 = Array Size(array=w352) -> (size(s)=w355:i32)
            n246 = case shown="默认" w355 {
              tunnel: w352 -> [w364 _]
              tunnel: w354 -> [w360 _]
              tunnel: [w359 w370] -> w353
              tunnel: w351 -> [w358 w371]
              frame Default {
                n247 = Index Array(array=w364, index=0) -> (element=w361:string)
                n248 = call "OpenDeviceBySN.vi"("error in (no error)"=w358, "SN"=w361, "IGxFactory"=w360) -> ("error out"=w357:errorcluster, "IGxDevice"=w362:refnum<k24>)
                n249 = case shown="无错误" w357 {
                  selector: w357 -> [w365 w368]
                  tunnel: w362 -> [w366 _]
                  tunnel: [w365 w368] -> w359
                  frame No Error {
                    n250 = local write "IGxDevice"(w366) -> ()
                    n251 = local write "设备状态"(TRUE) -> ()
                  }
                  frame Error {
                  }
                }
              }
              frame 0 {
                n252 = Merge Errors(w371, errorcluster {TRUE, 5001, "GxSingleCam.vi"}) -> (w370:errorcluster)
              }
            }
          }
          frame #1 {
            n253 = Generate User Event(user event=w372, event data cluster="UpdateParam") -> ()  [unwired: 2 in, 2 out]
            n254 = Generate User Event(user event=w372, event data cluster="PicShow") -> ()  [unwired: 2 in, 2 out]
          }
        }
      }
      event "关闭设备": Value Change {
        n255 = event-data() -> ()  [unwired: 1 in, 6 out]
        n256 = flat-sequence {
          tunnel: w376 -> [w381]
          tunnel: w377 -> [w406]
          frame #0 {
            n257 = local read "IGxStream"() -> (w385:refnum<k24>)
            n258 = local read "IGxDevice"() -> (w384:refnum<k24>)
            n259 = Not A Number/Path/Refnum?(number/path/refnum=w385) -> (NaN/Path/Refnum?=w386:bool)
            n260 = case shown="假" w386 {
              tunnel: w385 -> [w397 _]
              tunnel: w384 -> [w395 w405]
              tunnel: [w394 w405] -> w382
              tunnel: w381 -> [w392 _]
              frame False {
                n261 = call <vilib>:"Acquire Semaphore.vi"("semaphore"=w392) -> ("semaphore out"=w391:T2)  [unwired: 4 in, 2 out]
                n262 = flat-sequence {
                  tunnel: w397 -> [w399]
                  tunnel: [w400] -> w396
                  tunnel: w395 -> [w400]
                  tunnel: [w399] -> w393
                  tunnel: w391 -> [w398]
                  tunnel: [w398] -> w390
                  tunnel: w396 -> [w404]
                  tunnel: [w404] -> w394
                  tunnel: w393 -> [w402]
                  tunnel: [w401] -> w389
                  tunnel: w390 -> [w401]
                  frame #0 {
                    n263 = call "StopGrab.vi"("IGxStream"=w399, "IGxDevice"=w400) -> ()  [unwired: 1 in, 1 out]
                  }
                  frame #1 {
                    n264 = call "CloseStream.vi"("IGxStream"=w402) -> ("error out"=w403:errorcluster)  [unwired: 1 in]
                    n265 = Close Reference(reference=w402, error in (no error)=w403) -> ()  [unwired: 1 out]
                  }
                }
                n266 = call <vilib>:"Release Semaphore.vi"("semaphore"=w389) -> ()  [unwired: 5 in, 2 out]
              }
              frame True {
              }
            }
            n267 = local read "Image Src"() -> (w387:T1)
            n268 = call "CloseDevice.vi"("IGxDevice"=w382) -> ("error out"=w388:errorcluster)  [unwired: 1 in]
            n269 = Close Reference(reference=w382, error in (no error)=w388) -> (error out=w383:errorcluster)
            n270 = call "Imaq Dispose"("Image"=w387, "error in (no error)"=w383) -> ()  [unwired: 1 in, 4 out]
          }
          frame #1 {
            n271 = Generate User Event(user event=w406, event data cluster="UpdateUI") -> ()  [unwired: 2 in, 2 out]
          }
        }
        n272 = local write "采集状态"(FALSE) -> ()
        n273 = local write "设备状态"(FALSE) -> ()
      }
      event "开始采集": Value Change {
        n274 = event-data() -> ()  [unwired: 1 in, 6 out]
        n275 = flat-sequence {
          tunnel: [w414] -> w409
          tunnel: [w427] -> w410
          tunnel: w409 -> [w427]
          tunnel: w408 -> [w425]
          frame #0 {
            n276 = local read "IGxDevice"() -> (w417:refnum<k24>)
            n277 = call "OpenStream.vi"("StreamID"=0, "IGxDevice"=w417) -> ("error out"=w412:errorcluster, "IGxStream"=w415:refnum<k24>)  [unwired: 1 in]
            n278 = local write "IGxStream"(w415) -> ()
            n279 = call "StartGrab.vi"("error in (no error)"=w412, "IGxStream"=w415, "IGxDevice"=w417) -> ("error out"=w413:errorcluster)
            n280 = case shown="错误" w413 {
              selector: w413 -> [w418 w421]
              tunnel: w415 -> [_ w424]
              tunnel: [w418 w422] -> w414
              frame No Error {
                n281 = local write "采集状态"(TRUE) -> ()
              }
              frame Error {
                n282 = call "CloseStream.vi"("IGxStream"=w424) -> ("error out"=w423:errorcluster)  [unwired: 1 in]
                n283 = Close Reference(reference=w424, error in (no error)=w423) -> (error out=w420:errorcluster)
                n284 = Merge Errors(w421, w420) -> (w422:errorcluster)
              }
            }
          }
          frame #1 {
            n285 = Generate User Event(user event=w425, event data cluster="UpdateUI") -> ()  [unwired: 2 in, 2 out]
          }
        }
      }
      event "停止采集": Value Change {
        n286 = event-data() -> ()  [unwired: 1 in, 6 out]
        n287 = call <vilib>:"Acquire Semaphore.vi"("semaphore"=w436) -> ("semaphore out"=w432:T2)  [unwired: 4 in, 2 out]
        n288 = flat-sequence {
          tunnel: [w440] -> w434
          tunnel: w432 -> [w439]
          tunnel: [w439] -> w431
          tunnel: [w438] -> w428
          tunnel: [w444] -> w433
          tunnel: w434 -> [w446]
          tunnel: w431 -> [w443]
          tunnel: w428 -> [w442]
          tunnel: [w450] -> w429
          tunnel: w433 -> [w450]
          tunnel: w430 -> [w448]
          frame #0 {
            n289 = local read "IGxDevice"() -> (w441:refnum<k24>)
            n290 = local read "IGxStream"() -> (w440:refnum<k24>)
            n291 = call "StopGrab.vi"("IGxStream"=w440, "IGxDevice"=w441) -> ("error out"=w438:errorcluster)  [unwired: 1 in]
          }
          frame #1 {
            n292 = call "CloseStream.vi"("error in (no error)"=w442, "IGxStream"=w446) -> ("error out"=w447:errorcluster)
            n293 = Close Reference(reference=w446, error in (no error)=w447) -> (error out=w445:errorcluster)
            n294 = call <vilib>:"Release Semaphore.vi"("error in (no error)"=w445, "semaphore"=w443) -> ("error out"=w444:errorcluster)  [unwired: 4 in, 1 out]
          }
          frame #2 {
            n295 = Generate User Event(user event=w448, event data cluster="UpdateUI") -> ()  [unwired: 2 in, 2 out]
          }
        }
        n296 = local write "采集状态"(FALSE) -> ()
      }
      event "触发模式": Value Change {
        n297 = event-data() -> ()  [unwired: 1 in, 6 out]
        n298 = local read "IGxDevice"() -> (w458:refnum<k24>)
        n299 = local read "触发模式"() -> (w457:string)
        n300 = call "SetEnumValue.vi"("Enum Value"=w457, "Feature Name"="TriggerMode", "IGxDevice"=w458) -> ("error out"=w453:errorcluster)  [unwired: 1 in]
        n301 = Generate User Event(user event=w454, event data cluster="UpdateParam", error in=w453) -> (error out=w452:errorcluster)  [unwired: 1 in, 1 out]
      }
      event "触发源": Value Change {
        n302 = event-data() -> ()  [unwired: 1 in, 6 out]
        n303 = local read "IGxDevice"() -> (w466:refnum<k24>)
        n304 = local read "触发源"() -> (w464:string)
        n305 = call "SetEnumValue.vi"("Enum Value"=w464, "Feature Name"="TriggerSource", "IGxDevice"=w466) -> ("error out"=w462:errorcluster)  [unwired: 1 in]
        n306 = Generate User Event(user event=w461, event data cluster="UpdateUI", error in=w462) -> (error out=w460:errorcluster)  [unwired: 1 in, 1 out]
      }
      event "发送软触发": Value Change {
        n307 = event-data() -> ()  [unwired: 1 in, 6 out]
        n308 = local read "IGxDevice"() -> (w473:refnum<k24>)
        n309 = call "SetCommandValue.vi"("Feature Name"="TriggerSoftware", "IGxDevice"=w473) -> ("error out"=w470:errorcluster)  [unwired: 1 in]
        n310 = Generate User Event(user event=w469, event data cluster="UpdateUI", error in=w470) -> (error out=w467:errorcluster)  [unwired: 1 in, 1 out]
      }
      event "保存图片": Value Change {
        n311 = event-data() -> ()  [unwired: 1 in, 6 out]
        n312 = local read "保存图片"() -> (w475:bool)
        n313 = case shown="真" w475 {
          frame False {
          }
          frame True {
            n314 = call <vilib>:"Application Directory.vi"() -> ("Application Directory"=w482:path)
            n315 = Path To String(path=w482) -> (string=w481:string)
            n316 = Concatenate Strings(w481, "\\Image") -> (w479:string)
            n317 = String To Path(string=w479) -> (path=w477:path)
            n318 = call <vilib>:"Check if File or Folder Exists.vi"("path"=w477) -> ("file or folder exists?"=w478:bool)  [unwired: 8 in, 2 out]
            n319 = case shown="假" w478 {
              tunnel: w477 -> [w484 w485]
              tunnel: [w483 w485] -> w476
              frame False {
                n320 = Create Folder(path (use dialog)=w484) -> (created path=w483:path)  [unwired: 2 in, 2 out]
              }
              frame True {
              }
            }
            n321 = local write "图片存储路径"(w476) -> ()
          }
        }
      }
      event "安全退出": Value Change {
        n322 = event-data() -> ()  [unwired: 1 in, 6 out]
        n323 = flat-sequence {
          tunnel: w486 -> [w489]
          tunnel: w487 -> [w517]
          frame #0 {
            n324 = local read "采集状态"() -> (w492:bool)
            n325 = local read "IGxDevice"() -> (w491:refnum<k24>)
            n326 = local read "IGxStream"() -> (w493:refnum<k24>)
            n327 = case shown="真" w492 {
              tunnel: w493 -> [_ w507]
              tunnel: w491 -> [w498 w506]
              tunnel: [w498 w504] -> w490
              tunnel: w489 -> [_ w502]
              frame False {
              }
              frame True {
                n328 = call <vilib>:"Acquire Semaphore.vi"("semaphore"=w502) -> ("semaphore out"=w501:T2)  [unwired: 4 in, 2 out]
                n329 = flat-sequence {
                  tunnel: w507 -> [w509]
                  tunnel: w506 -> [w510]
                  tunnel: [w510] -> w505
                  tunnel: [w509] -> w503
                  tunnel: w501 -> [w508]
                  tunnel: [w508] -> w500
                  tunnel: [w515] -> w504
                  tunnel: w505 -> [w515]
                  tunnel: w503 -> [w513]
                  tunnel: [w511] -> w499
                  tunnel: w500 -> [w511]
                  frame #0 {
                    n330 = call "StopGrab.vi"("IGxStream"=w509, "IGxDevice"=w510) -> ()  [unwired: 1 in, 1 out]
                  }
                  frame #1 {
                    n331 = local write "采集状态"(FALSE) -> ()
                    n332 = call "CloseStream.vi"() -> ("error out"=w514:errorcluster)  [unwired: 2 in]
                    n333 = Close Reference(reference=w513, error in (no error)=w514) -> ()  [unwired: 1 out]
                  }
                }
                n334 = call <vilib>:"Release Semaphore.vi"("semaphore"=w499) -> ()  [unwired: 5 in, 2 out]
              }
            }
            n335 = local read "设备状态"() -> (w494:bool)
            n336 = case shown="真" w494 {
              tunnel: w490 -> [_ w495]
              frame False {
              }
              frame True {
                n337 = call "CloseDevice.vi"("IGxDevice"=w495) -> ("error out"=w497:errorcluster)  [unwired: 1 in]
                n338 = local write "设备状态"(FALSE) -> ()
                n339 = Close Reference(reference=w495, error in (no error)=w497) -> ()  [unwired: 1 out]
              }
            }
          }
          frame #1 {
            n340 = local write "是否退出"(TRUE) -> ()
            n341 = Generate User Event(user event=w517, event data cluster="Quit") -> ()  [unwired: 2 in, 2 out]
          }
        }
      }
      event Panel Close? {
        n342 = event-data() -> ()  [unwired: 1 in, 4 out]
        n343 = flat-sequence {
          tunnel: w519 -> [w522]
          tunnel: w520 -> [w549]
          frame #0 {
            n344 = local read "采集状态"() -> (w525:bool)
            n345 = local read "IGxDevice"() -> (w524:refnum<k24>)
            n346 = local read "IGxStream"() -> (w526:refnum<k24>)
            n347 = case shown="真" w525 {
              tunnel: w526 -> [_ w540]
              tunnel: w524 -> [w531 w539]
              tunnel: [w531 w537] -> w523
              tunnel: w522 -> [_ w535]
              frame False {
              }
              frame True {
                n348 = call <vilib>:"Acquire Semaphore.vi"("semaphore"=w535) -> ("semaphore out"=w534:T2)  [unwired: 4 in, 2 out]
                n349 = flat-sequence {
                  tunnel: w540 -> [w542]
                  tunnel: w539 -> [w543]
                  tunnel: [w543] -> w538
                  tunnel: [w542] -> w536
                  tunnel: w534 -> [w541]
                  tunnel: [w541] -> w533
                  tunnel: [w548] -> w537
                  tunnel: w538 -> [w548]
                  tunnel: w536 -> [w546]
                  tunnel: [w544] -> w532
                  tunnel: w533 -> [w544]
                  frame #0 {
                    n350 = call "StopGrab.vi"("IGxStream"=w542, "IGxDevice"=w543) -> ()  [unwired: 1 in, 1 out]
                  }
                  frame #1 {
                    n351 = local write "采集状态"(FALSE) -> ()
                    n352 = call "CloseStream.vi"() -> ("error out"=w547:errorcluster)  [unwired: 2 in]
                    n353 = Close Reference(reference=w546, error in (no error)=w547) -> ()  [unwired: 1 out]
                  }
                }
                n354 = call <vilib>:"Release Semaphore.vi"("semaphore"=w532) -> ()  [unwired: 5 in, 2 out]
              }
            }
            n355 = local read "设备状态"() -> (w527:bool)
            n356 = case shown="真" w527 {
              tunnel: w523 -> [_ w528]
              frame False {
              }
              frame True {
                n357 = call "CloseDevice.vi"("IGxDevice"=w528) -> ("error out"=w530:errorcluster)  [unwired: 1 in]
                n358 = local write "设备状态"(FALSE) -> ()
                n359 = Close Reference(reference=w528, error in (no error)=w530) -> ()  [unwired: 1 out]
              }
            }
          }
          frame #1 {
            n360 = local write "是否退出"(TRUE) -> ()
            n361 = Generate User Event(user event=w549, event data cluster="Quit") -> ()  [unwired: 2 in, 2 out]
          }
        }
        n362 = event-data() -> ()  [unwired: 2 in, 1 out]
      }
    }
    "error out" <- w343
    n363 = call <vilib>:"Simple Error Handler.vi"("error in (no error)"=w343) -> ()  [unwired: 4 in, 5 out]
  }
  n364 = Stop(stop? (T)=w3) -> ()
